vi "initialise.vi"(8 "error in (no error)":errorcluster, 11 "GenericPlugin in":refnum<class "TrajectoryAK101022Resonance.lvclass">) -> (0 "error out":errorcluster, 3 "GenericPlugin out":refnum<class "TrajectoryAK101022Resonance.lvclass">)   [LabVIEW 2010, in "TrajectoryAK101022Resonance.lvclass"]
doc: "The dynamic dispatch-version of this VI initalises the plug-in object by allocating and initalising any dynamic resources need."
uses:
  TrajectoryAK101022Resonance.lvclass
  TrajectoryMG100122GenericFPGA/TrajectoryMG100122GenericFPGA/TrajectoryMG100122GenericFPGA.lvclass
  TrajectoryAK101022Resonance.lvclass/TrajectoryAK101022Resonance.ctl
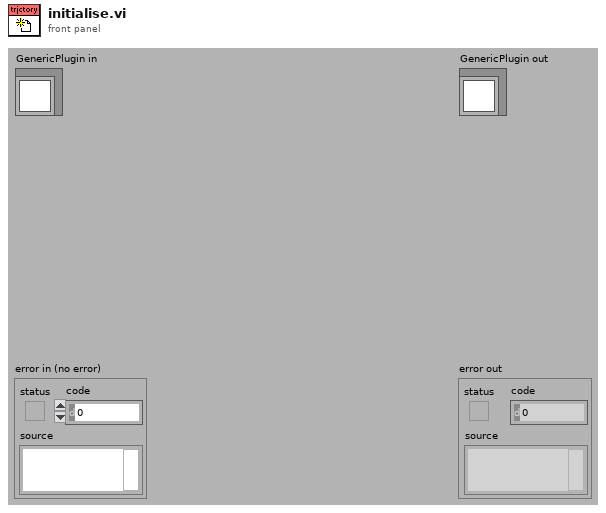
[diagram p1: front panel]
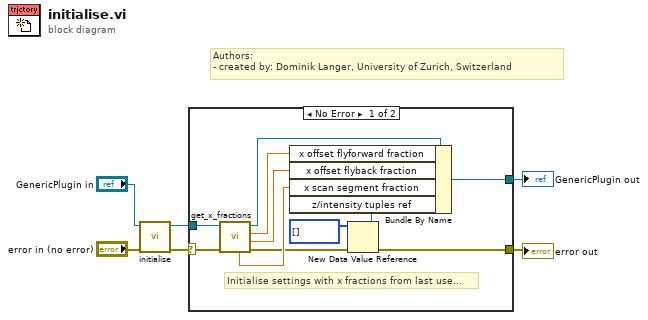
[diagram p0: block diagram]
diagram:
  # "Authors: \n- created by: Dominik Langer, University of Zurich, Switzerland"
  n1 = call-parent "initialise.vi"("error in (no error)"="error in (no error)", "GenericPlugin in"="GenericPlugin in") -> ("error out"=w3:errorcluster, "GenericPlugin out"=w4:refnum<class "TrajectoryAK101022Resonance.lvclass">)  [unwired: 8 in]
  n2 = case shown="No Error" w3 {
    selector: w3 -> [w16 w18]
    tunnel: w4 -> [w17 w19]
    tunnel: [w8 w18] -> w2
    tunnel: [w13 w19] -> w1
    frame No Error {
      # "Initialise settings with x fractions from last use..."
      n3 = call "get_x_fractions.vi"("error in (no error)"=w16, "TrajectoryAK101022Resonance in"=w17) -> ("error out"=w9:errorcluster, "x offset fly back fraction"=w12:dbl, "x offset fly forward fraction"=w14:dbl, "TrajectoryAK101022Resonance out"=w15:refnum<class "TrajectoryAK101022Resonance.lvclass">, "x scan segment fraction"=w11:dbl)  [unwired: 5 in]
      n4 = New Data Value Reference(data value=u32[] [], error in=w9) -> (data value reference=w7:refnum<data-value>, error out=w8:errorcluster)
      n5 = Bundle By Name(cluster=w15, "x offset flyforward fraction"=w14, "x offset flyback fraction"=w12, "x scan segment fraction"=w11, "z/intensity tuples ref"=w7) -> (w13:refnum<class "TrajectoryAK101022Resonance.lvclass">)
    }
    frame Error {
    }
  }
  "error out" <- w2
  "GenericPlugin out" <- w1
